vi "Q Vision_Color to RGB.vi"(0 "Color":u32(colorbox)) -> (14 "RGB":u8[](array[numeric]))   [LabVIEW 2016]
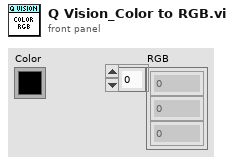
[diagram p1: front panel]
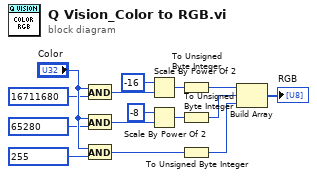
[diagram p0: block diagram]
diagram:
  n1 = And(x="Color", y=u32 16711680) -> (x .and. y?=w13:u32)
  n2 = And(x="Color", y=u32 65280) -> (x .and. y?=w14:u32)
  n3 = And(x="Color", y=u32 255) -> (x .and. y?=w5:u32)
  n4 = Scale By Power Of 2(n=i16 -16, x=w13) -> (x*2^n=w7:u32)
  n5 = Scale By Power Of 2(n=i16 -8, x=w14) -> (x*2^n=w6:u32)
  n6 = To Unsigned Byte Integer(number=w7) -> (unsigned 8bit integer=w4:u8)
  n7 = To Unsigned Byte Integer(number=w6) -> (unsigned 8bit integer=w3:u8)
  n8 = To Unsigned Byte Integer(number=w5) -> (unsigned 8bit integer=w2:u8)
  n9 = Build Array(w4, w3, w2) -> (→"RGB":u8[])
